vi "MethodCall.vi"(8 "error in":errorcluster, 9 "Method Params":string[](array[string]), 10 "methodName":string="getParam", 11 "Node ROS":T1={"topic port"=0, "Node"="", "topic"="", "type"="", "node port"=0, "error "={"status"=FALSE, "code"=0, "source"=""}, "Direction"=enum."Node", "APIs"=[], "Update (ms)"=1, "write queue"=1}) -> (0 "error out":errorcluster, 3 "XML Received":string)   [LabVIEW 2012]
uses:
  <userlib>/ROSforLV/ROS/Code/SubVIs/_ROSControl.ctl
  <userlib>/ROSforLV/ROS/Code/SubVIs/_ROSDirection.ctl
  <userlib>/ROSforLV/ROS/Code/_ROSDefinition.vi
panel:
  out "XML Sent":string
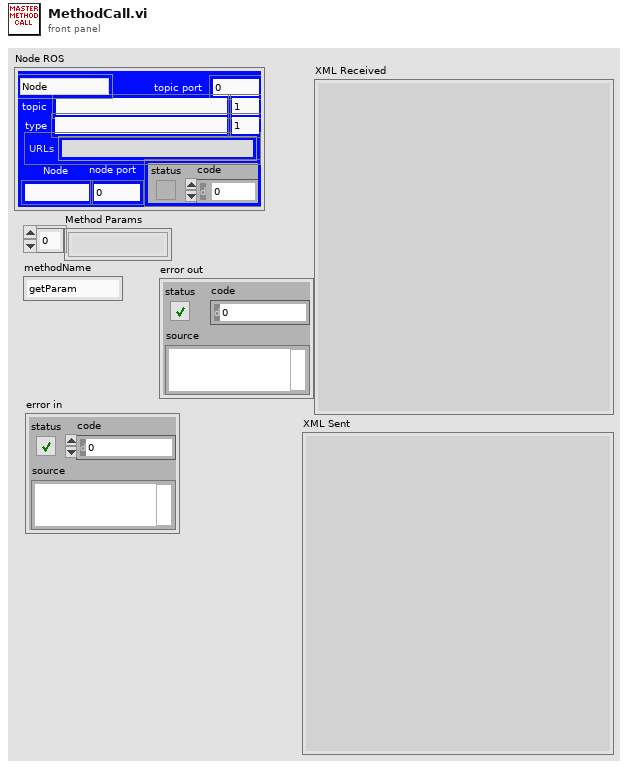
[diagram p1: front panel]
types:
  T1 = typedef "_ROSControl.ctl" = cluster{"topic port":u16, "Node":string, "topic":string, "type":string, "node port":u32, "error ":errorcluster, "Direction":T2, "APIs":string[], "Update (ms)":u16, "write queue":u16}
  T2 = typedef "_ROSDirection.ctl" = enum16{"Node", "Publisher", "Subscriber", "Service Client"}
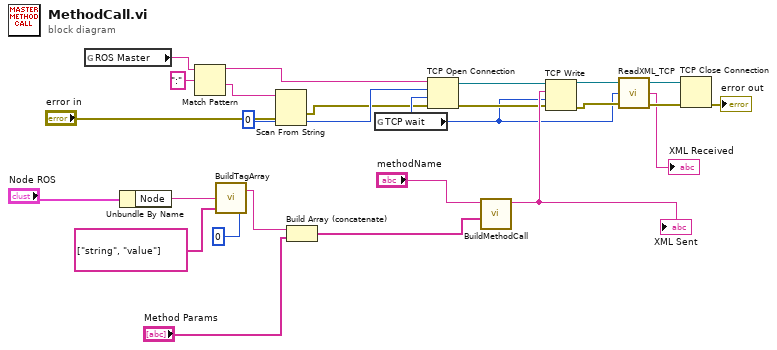
[diagram p0: block diagram]
diagram:
  n1 = global read "_ROSDefinition.vi" "ROS Master"() -> (w9:string)
  n2 = Unbundle By Name("Node ROS") -> ("Node"=w5:string)
  n3 = Match Pattern(string=w9, regular expression=":") -> (before substring=w10:string, after substring=w7:string)  [unwired: 1 in, 2 out]
  n4 = call <userlib>:"BuildTagArray.vi"("Indent"=i8 0, "tags"=string[] ["string", "value"], "value"=w5) -> ("string out"=w24:string)  [unwired: 1 in]
  n5 = Scan From String(input string=w7, error in="error in", default 1=u16 0 ("remote port or service name")) -> (error out=w1:errorcluster, output 1=w11:u16)  [unwired: 2 in, 2 out]
  n6 = Build Array (concatenate)(w24, "Method Params") -> (w23:string[])
  n7 = global read "_ROSDefinition.vi" "TCP wait"() -> (w17:i32)
  n8 = TCP Open Connection(address=w10, remote port or service name=w11, timeout ms (60000)=w17, error in (no error)=w1) -> (connection ID=w19:refnum<k5>, error out=w18:errorcluster)  [unwired: 1 in]
  n9 = call <userlib>:"BuildMethodCall.vi"("params"=w23, "methodName"="methodName") -> ("XML"=w22:string)  [unwired: 9 in]
  "XML Sent" <- w22
  n10 = TCP Write(connection ID=w19, data in=w22, error in (no error)=w18, 9:w17) -> (connection ID out=w20:refnum<k5>, error out=w21:errorcluster)  [unwired: 1 out]
  n11 = call <userlib>:"ReadXML_TCP.vi"("error in"=w21, "timeout ms (3000)"=w17, "connection ID in"=w20) -> ("error out"=w15:errorcluster, "data out"=→"XML Received":string, "connection ID out"=w16:refnum<k5>)
  n12 = TCP Close Connection(connection ID=w16, error in (no error)=w15) -> (error out=→"error out":errorcluster)  [unwired: 1 in, 1 out]
